vi "Write Register.vi"(8 "error in (no error)":errorcluster, 9 "Data":u8 format="%.0x", 10 "Register Address":u8 format="%.0x", 11 "LINX-ADS1256 in":refnum<class "LINX-ADS1256.lvclass">) -> (0 "error out":errorcluster, 3 "LINX-ADS1256 out":refnum<class "LINX-ADS1256.lvclass">)   [LabVIEW 2020, in "LINX-ADS1256.lvclass"]
doc: "Writes data to the register at the given address."
uses:
  LINX-ADS1256.lvclass
  LINX SPI/LINX SPI.lvclass
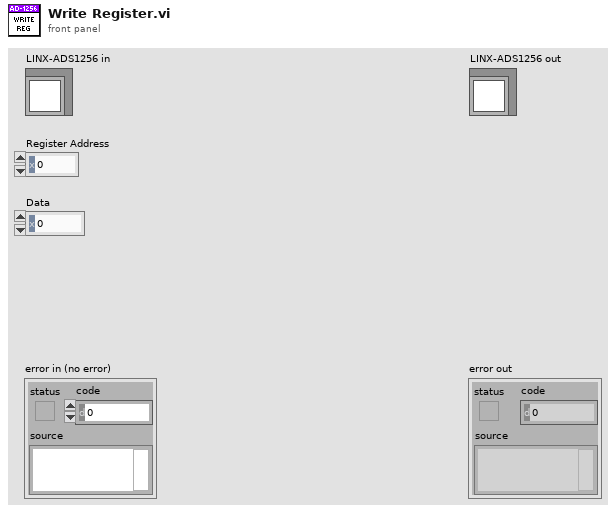
[diagram p1: front panel]
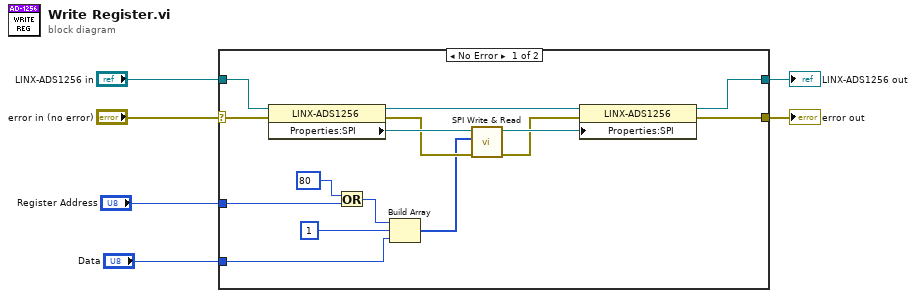
[diagram p0: block diagram]
diagram:
  n1 = case shown="No Error" "error in (no error)" {
    selector: "error in (no error)" -> [w14 w23]
    tunnel: [w13 w23] -> w5
    tunnel: [w15 w22] -> w3
    tunnel: "LINX-ADS1256 in" -> [w21 w22]
    tunnel: "Register Address" -> [w12 _]
    tunnel: "Data" -> [w7 _]
    frame No Error {
      n2 = property class="LINX-ADS1256"(reference=w21, error in=w14) -> (reference out=w17:refnum<class "LINX-ADS1256.lvclass">, error out=w18:errorcluster, "Properties:SPI"=w20:refnum<class "LINX SPI.lvclass">)
      n3 = Or(x=u8 80 ("SPI Channel"), y=w12) -> (x .or. y?=w10:u8)
      n4 = Build Array(w10, u8 1 ("SPI Channel"), w7) -> (w8:u8[])
      n5 = call "SPI Write & Read.vi"("error in (no error)"=w18, "Data"=w8, "LINX SPI in"=w20) -> ("error out"=w16:errorcluster, "LINX SPI out"=w19:refnum<class "LINX SPI.lvclass">)  [unwired: 6 in, 1 out]
      n6 = property class="LINX-ADS1256"(reference=w17, error in=w16, "Properties:SPI"=w19) -> (reference out=w15:refnum<class "LINX-ADS1256.lvclass">, error out=w13:errorcluster)
    }
    frame Error {
    }
  }
  "error out" <- w5
  "LINX-ADS1256 out" <- w3
